vi "Load-Settings.vi"() -> ()   [LabVIEW 2017]
uses:
  Settings-Control.ctl
  Traverse-Settings-Global.vi
panel:
  in  "Settings":T1
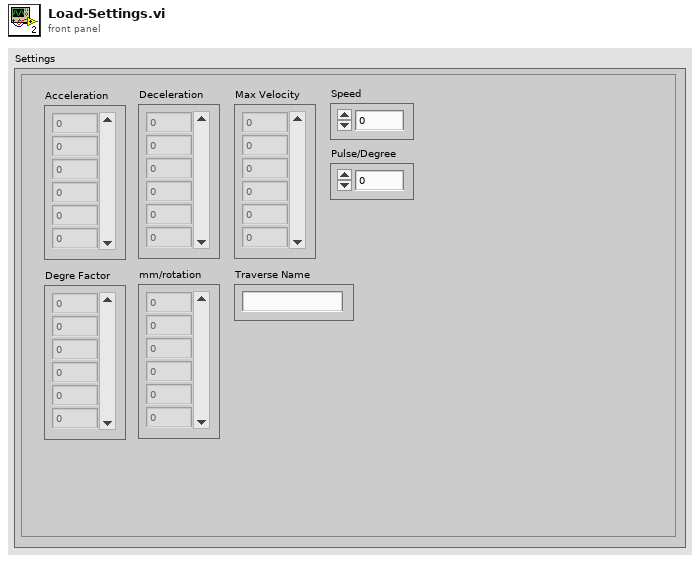
[diagram p1: front panel]
types:
  T1 = typedef "Settings-Control.ctl" = cluster{"Acceleration":dbl[], "Deceleration":dbl[], "Max Velocity":dbl[], "Speed":dbl, "Pulse/Degree":dbl, "Degre Factor":dbl[], "mm/rotation":dbl[], "Traverse Name":string}
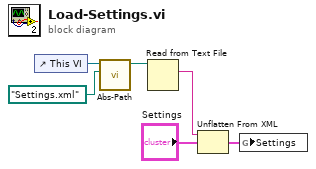
[diagram p0: block diagram]
diagram:
  n1 = control-ref of="This VI"() -> (w4:refnum<vi>)
  n2 = call "Abs-Path.vi"("filename"=path "Settings.xml" ("file (use dialog)"), "Vi in path"=w4) -> ("Full path"=w3:path)  [unwired: 9 in]
  n3 = Read from Text File(file (use dialog)=w3) -> (text=w6:string)  [unwired: 3 in, 3 out]
  n4 = Unflatten From XML(xml string=w6, type="Settings") -> (value=w2:T1)  [unwired: 1 in, 1 out]
  n5 = global write "Traverse-Settings-Global.vi" "Settings"(w2) -> ()
